vi "thermal_optical_camera_3.vi"() -> ()   [LabVIEW 2025]
panel:
  in  "Stop (F)":bool
  in  "Acquisition Control:\nExposure Time [100, 3E7]":dbl=999.0 caption="Acquisition Control::Exposure Time" min=100.0 max=29999995.0
  in  "Analog Control:\nGain [0, 27]":dbl caption="Analog Control::Gain" min=0.0 max=27.045663671679687
  in  "Analog Control:\nBlack Level [-5, 10]":dbl caption="Analog Control::Black Level" min=-5.0000011920928955 max=10.000002384185791
  in  "Analog Control:\nGamma [0.25, 4.00]":dbl=0.800048828125 caption="Analog Control::Gamma" min=0.25 max=4.0 step=0.05
  out "Optical camera":T1(plugin-control)
  in  "optical capture interval (s)":dbl
  in  "File Path":string="C:\\Digambar\\Metal_thin_wall\\Optical_images\\Optical_images"
  out "File Name Out":string
  out "Frames":i32
  in  "thermal capture interval (s)":dbl
  out "Thermal camera":T1(plugin-control)
  out "Output":string
  in  "Flag Button":bool
  in  "Stop & Save":bool
  in  "Stop Preview":bool
  in  "Focus":dbl(slide) scale=0.0..100.0
  in  "Record":bool
  # "(1) Run VI"
  # "(2) After thermal camera calibration message (in terminal), press START"
  # "(3) Stop & Save"
  # "Destination for Optical Images:"
  # "(Enter \"28\")"
  # "Thermal Record"
  # "change folder names each time you run,\nso it saves data sets in dedicated folders:\nfolder1\nfolder2\nfolder3\netc..."
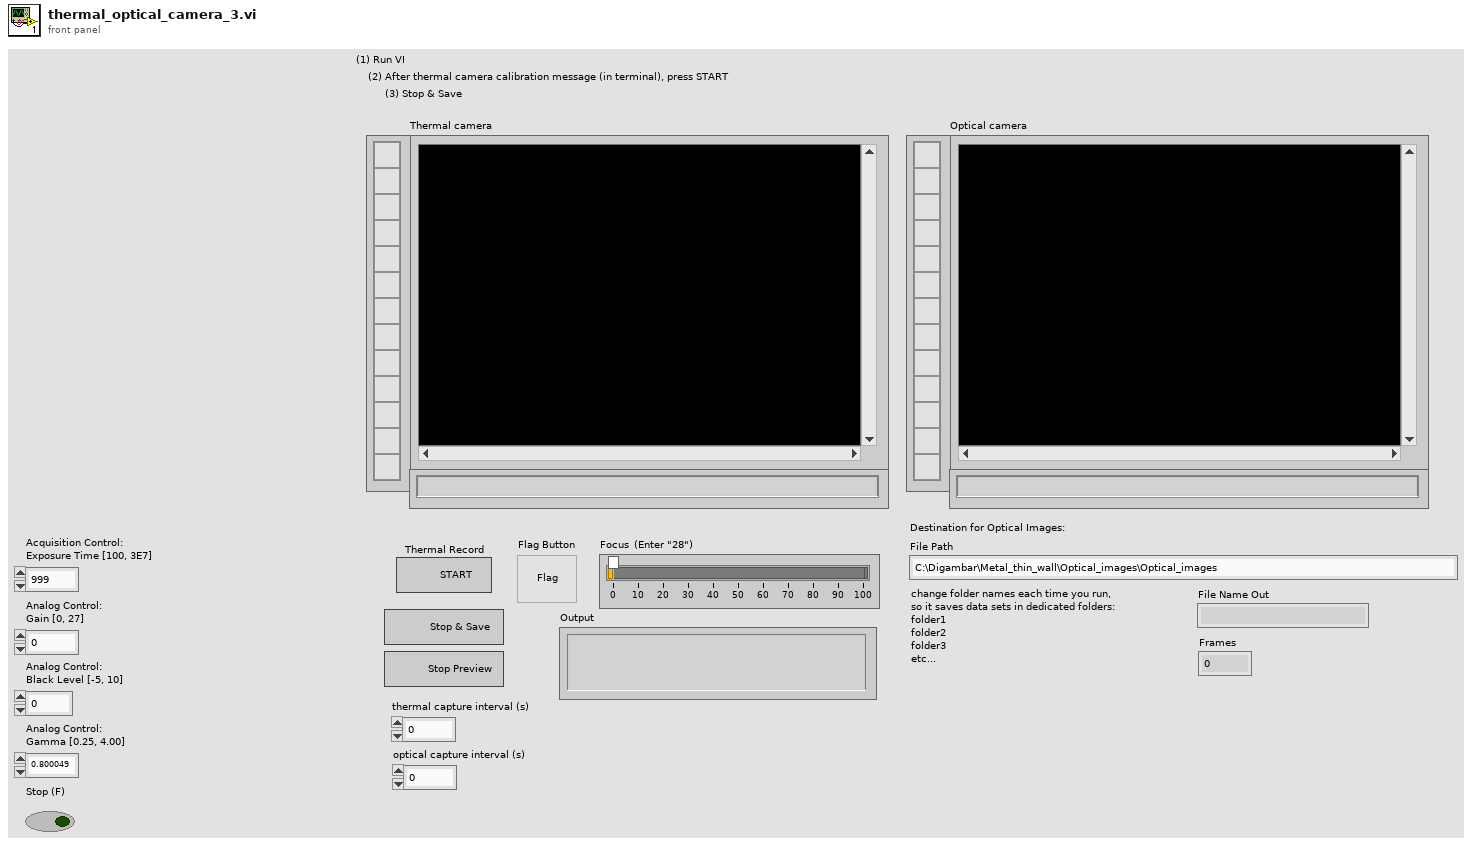
[diagram p1: front panel]
types:
  T1 = typedef "IMAQ Image.ctl" = refnum<image>
  T2 = enum16{"Standard", "Buffered", "CRLF", "Immediate"}
  T3 = enum16{"open", "replace", "create", "open or create", "replace or create", "replace or create with confirmation"}
  T4 = enum16{"big-endian, network order", "native, host order", "little-endian"}
  T5 = typedef "Image Type" = u32
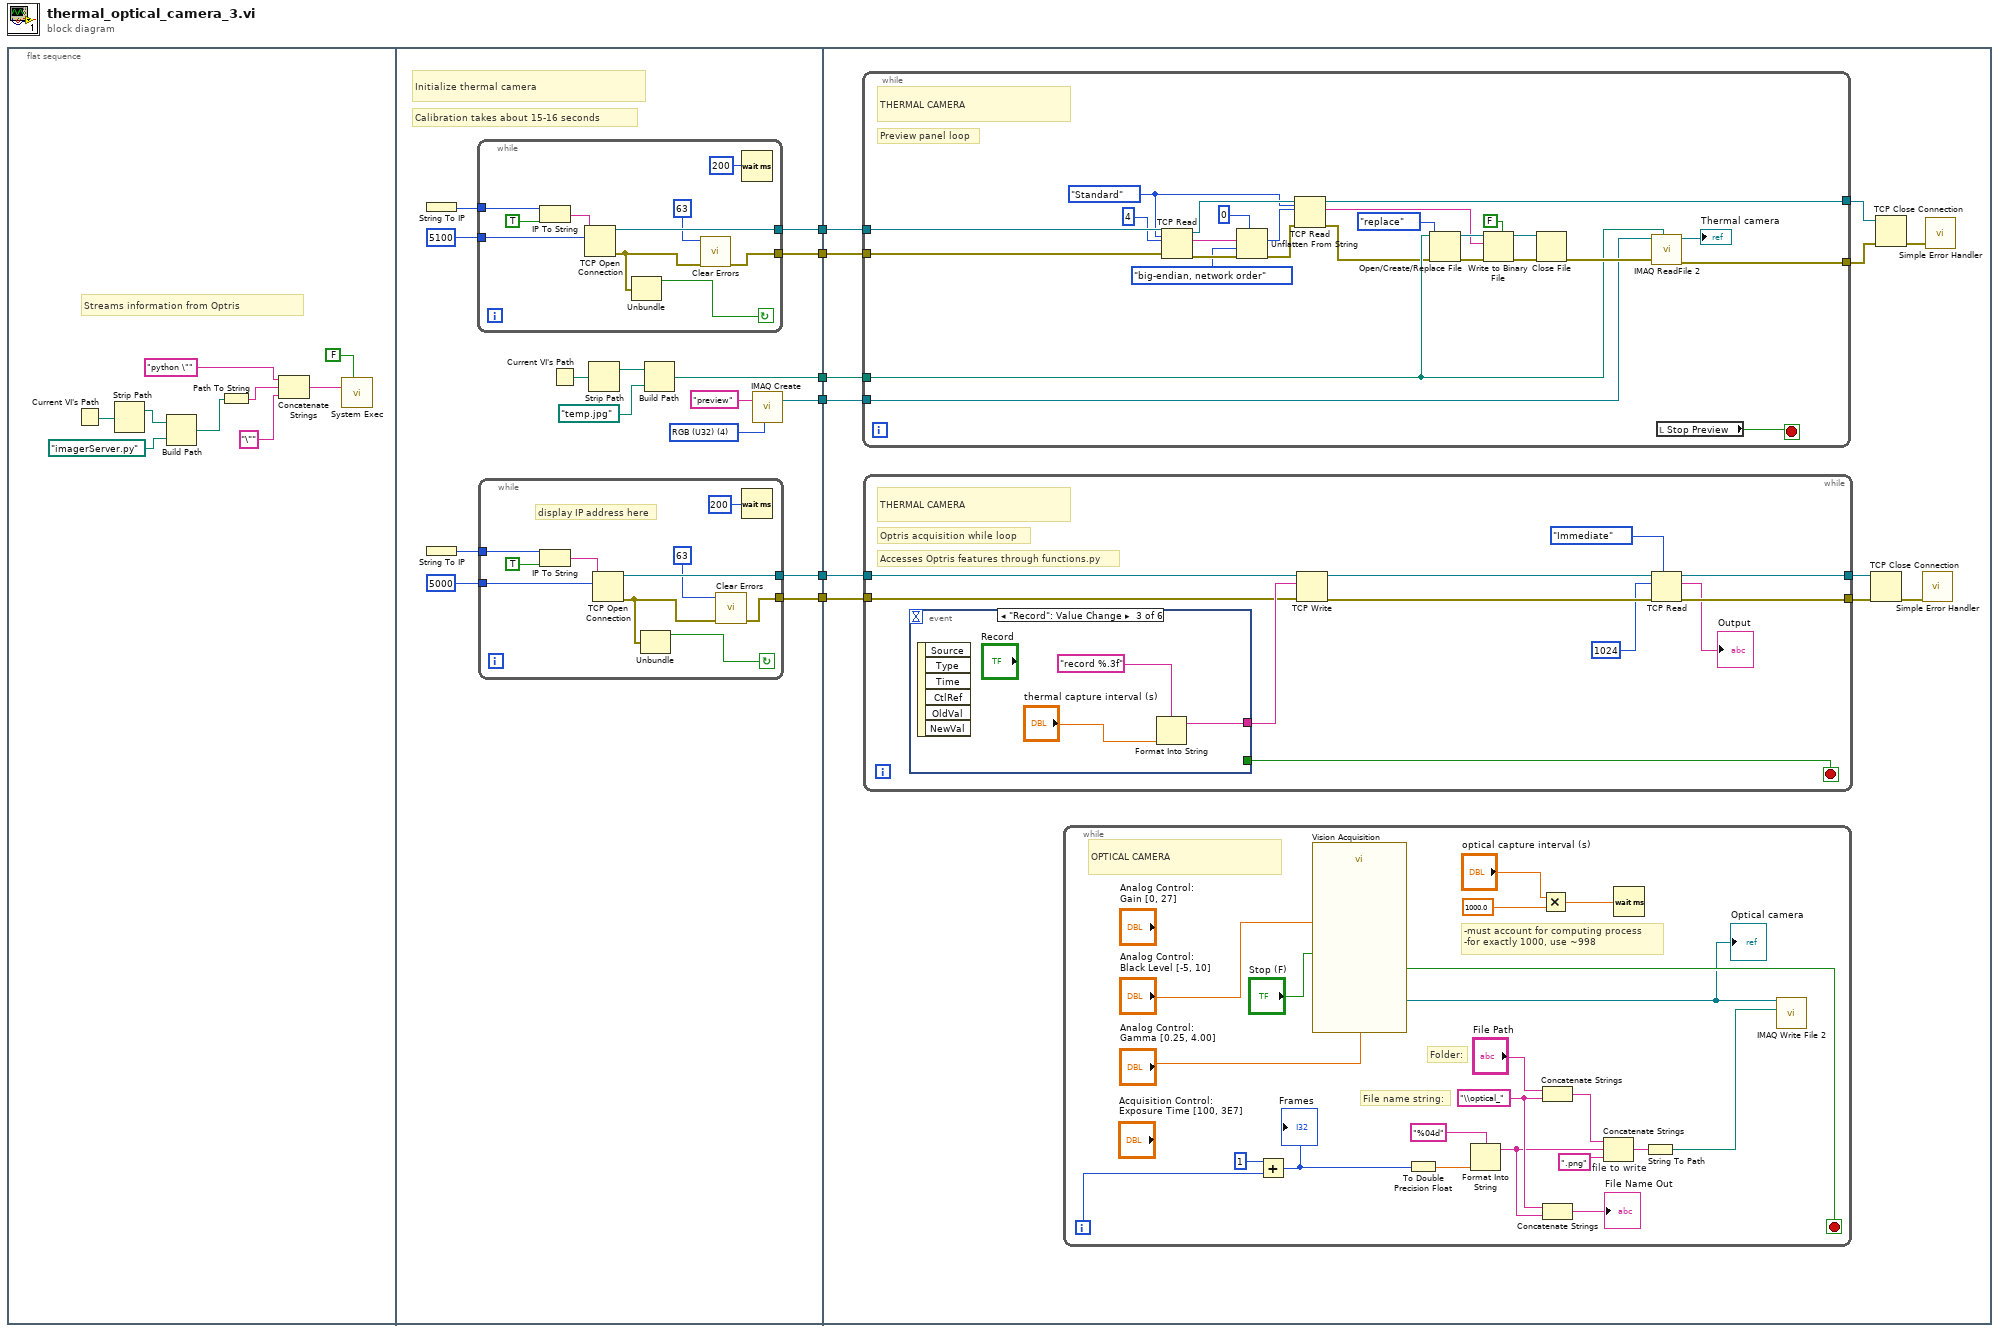
[diagram p0: block diagram]
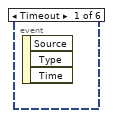
[diagram p2: hidden frame]
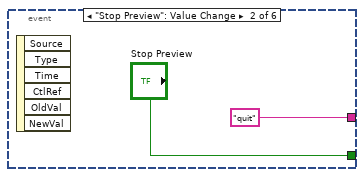
[diagram p3: hidden frame]
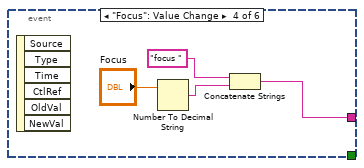
[diagram p4: hidden frame]
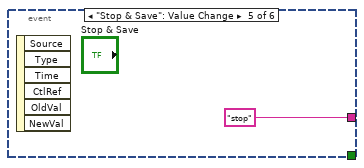
[diagram p5: hidden frame]
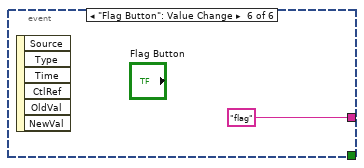
[diagram p6: hidden frame]
diagram:
  n1 = flat-sequence {
    tunnel: [w21] -> w6
    tunnel: [w20] -> w5
    tunnel: [w19] -> w4
    tunnel: [w18] -> w3
    tunnel: [w17] -> w2
    tunnel: [w16] -> w1
    tunnel: w1 -> [w56]
    tunnel: w2 -> [w57]
    tunnel: w3 -> [w52]
    tunnel: w4 -> [w51]
    tunnel: w5 -> [w58]
    tunnel: w6 -> [w59]
    frame #0 {
      # "Streams information from Optris"
      n2 = Current VI's Path() -> (path=w10:path)
      n3 = Strip Path(path=w10) -> (stripped path=w11:path)  [unwired: 1 out]
      n4 = Build Path(base path=w11, name or relative path=path "imagerServer.py") -> (appended path=w8:path)
      n5 = Path To String(path=w8) -> (string=w14:string)
      n6 = Concatenate Strings("python \"" ("string"), w14, "\"" ("string")) -> (w13:string)
      n7 = call <vilib>:"System Exec.vi"("wait until completion? (T)"=FALSE, "command line"=w13) -> ()  [unwired: 6 in, 4 out]
    }
    frame #1 {
      w22 = T5 4 items=["Grayscale (U8)", "Grayscale (I16)", "Grayscale (SGL)", "Complex (CSG)", "RGB (U32)", "HSL (U32)", "RGB (U64)", "Grayscale (U16)"] ("Image Type")
      # "Initialize thermal camera"
      # "Calibration takes about 15-16 seconds"
      n8 = String To IP() -> (0:w30:u32)  [unwired: 1 in]
      n9 = String To IP() -> (0:w29:u32)  [unwired: 1 in]
      n10 = while {
        tunnel: w30 -> [w40]
        tunnel: [w34] -> w21
        tunnel: [w38] -> w20
        tunnel: u16 5100 ("remote port or service name") -> [w36]
        stop <- w31 continue-if-true
        n11 = IP To String(1:TRUE ("dot notation? (F)"), 2:w40) -> (0:w39:string)
        n12 = TCP Open Connection(address=w39, remote port or service name=w36) -> (connection ID=w38:refnum<k5>, error out=w35:errorcluster)  [unwired: 3 in]
        n13 = Unbundle(w35) -> ("status"=w31:bool)  [unwired: 2 out]
        n14 = call <vilib>:"Clear Errors.vi"("error in (no error)"=w35, "specific error code to clear (0: all)"=63) -> ("error out"=w34:errorcluster)  [unwired: 4 in, 1 out]
        n15 = Wait (ms)(milliseconds to wait=u32 200) -> ()  [unwired: 1 out]
      }
      n16 = while {
        tunnel: [w44] -> w19
        tunnel: [w50] -> w18
        tunnel: w29 -> [w48]
        tunnel: u16 5000 ("remote port or service name") -> [w46]
        stop <- w41 continue-if-true
        # "display IP address here"
        n17 = IP To String(1:TRUE ("dot notation? (F)"), 2:w48) -> (0:w49:string)
        n18 = TCP Open Connection(address=w49, remote port or service name=w46) -> (connection ID=w50:refnum<k5>, error out=w45:errorcluster)  [unwired: 3 in]
        n19 = Unbundle(w45) -> ("status"=w41:bool)  [unwired: 2 out]
        n20 = call <vilib>:"Clear Errors.vi"("error in (no error)"=w45, "specific error code to clear (0: all)"=63) -> ("error out"=w44:errorcluster)  [unwired: 4 in, 1 out]
        n21 = Wait (ms)(milliseconds to wait=u32 200) -> ()  [unwired: 1 out]
      }
      n22 = Current VI's Path() -> (path=w28:path)
      n23 = Strip Path(path=w28) -> (stripped path=w27:path)  [unwired: 1 out]
      n24 = Build Path(base path=w27, name or relative path=path "temp.jpg") -> (appended path=w17:path)
      n25 = call "IMAQ Create"("Image Name"="preview", "Image Type"=w22) -> ("New Image"=w16:T1)  [unwired: 3 in, 1 out]
    }
    frame #2 {
      n26 = while {
        tunnel: [w129] -> w61
        tunnel: [w131] -> w62
        tunnel: w59 -> [w126]
        tunnel: w58 -> [w125]
        tunnel: w57 -> [w128]
        tunnel: w56 -> [w124]
        stop <- w127 stop-if-true
        w116 = T2."Standard" ("mode (standard)")
        # "THERMAL CAMERA"
        # "Preview panel loop"
        n27 = TCP Read(connection ID=w125, bytes to read=4, error in (no error)=w126, 7:w116) -> (connection ID out=w119:refnum<k5>, data out=w107:string, error out=w122:errorcluster)  [unwired: 1 in]
        n28 = Unflatten From String(type=0, binary string=w107, byte order (0:big-endian, network order)=T4."big-endian, network order", error in (no error)=w122) -> (value=w117:i32, error out=w118:errorcluster)  [unwired: 1 in, 1 out]
        n29 = TCP Read(connection ID=w119, bytes to read=w117, error in (no error)=w118, 7:w116) -> (connection ID out=w131:refnum<k5>, data out=w112:string, error out=w114:errorcluster)  [unwired: 1 in]
        n30 = Open/Create/Replace File(file path (use dialog)=w128, error in=w114, operation (0:open)=T3."replace") -> (refnum out=w113:refnum<file>, error out=w110:errorcluster)  [unwired: 3 in, 1 out]
        n31 = Write to Binary File(file (use dialog)=w113, data=w112, error in=w110, 5:FALSE ("prepend array or string size? (T)")) -> (refnum out=w108:refnum<file>, error out=w109:errorcluster)  [unwired: 2 in, 1 out]
        n32 = Close File(refnum=w108, error in=w109) -> (error out=w130:errorcluster)  [unwired: 1 out]
        n33 = call "IMAQ ReadFile 2"("File Path"=w128, "error in (no error)"=w130, "Image"=w124) -> ("error out"=w129:errorcluster, "Image Out"=→"Thermal camera":T1)  [unwired: 4 in, 3 out]
        n34 = local read "Stop Preview"() -> (w127:bool)
      }
      n35 = while {
        tunnel: [w93] -> w53
        tunnel: [w91] -> w54
        tunnel: w52 -> [w85]
        tunnel: w51 -> [w84]
        stop <- w86 stop-if-true
        # "THERMAL CAMERA"
        # "Optris acquisition while loop"
        # "Accesses Optris features through functions.py"
        n36 = event shown="[2] \"Record\": Value Change" {
          selector: _ -> [_ _ _ _ _ _]
          dyn-events: _ -> [_ _ _ _ _ _]
          timeout: _ -> [_ _ _ _ _ _]
          tunnel: [_ "quit" w99 w101 "stop" "flag"] -> w90
          tunnel: [_ "Stop Preview" _ _ _ _] -> w86
          event Timeout {
            n37 = event-data() -> ()  [unwired: 1 in, 3 out]
          }
          event "Stop Preview": Value Change {
            n38 = event-data() -> ()  [unwired: 1 in, 6 out]
          }
          event "Record": Value Change {
            n39 = event-data() -> ()  [unwired: 1 in, 6 out]
            n40 = Format Into String(format string="record %.3f", "thermal capture interval (s)") -> (resulting string=w99:string)  [unwired: 2 in, 1 out]
          }
          event "Focus": Value Change {
            n41 = event-data() -> ()  [unwired: 1 in, 6 out]
            n42 = Number To Decimal String(number="Focus") -> (decimal integer string=w103:string)  [unwired: 1 in]
            n43 = Concatenate Strings("focus ", w103) -> (w101:string)
          }
          event "Stop & Save": Value Change {
            n44 = event-data() -> ()  [unwired: 1 in, 6 out]
          }
          event "Flag Button": Value Change {
            n45 = event-data() -> ()  [unwired: 1 in, 6 out]
          }
        }
        n46 = TCP Write(connection ID=w85, data in=w90, error in (no error)=w84) -> (connection ID out=w92:refnum<k5>, error out=w94:errorcluster)  [unwired: 1 in, 1 out]
        n47 = TCP Read(connection ID=w92, bytes to read=1024, error in (no error)=w94, 7:T2."Immediate" ("mode (standard)")) -> (connection ID out=w91:refnum<k5>, data out=→"Output":string, error out=w93:errorcluster)  [unwired: 1 in]
      }
      n48 = while {
        i -> [w64]
        stop <- w82 stop-if-true
        w70 = "\\optical_" ("string")
        # "-must account for computing process\n-for exactly 1000, use ~998"
        # "OPTICAL CAMERA"
        # "Folder:"
        # "File name string:"
        n49 = Add(x=1, y=w64) -> (x+y=w63:i32)
        "Frames" <- w63
        n50 = call "Vision Acquisition"("Analog Control::Black Level"="Analog Control:\nBlack Level [-5, 10]", "Analog Control::Gamma"="Analog Control:\nGamma [0.25, 4.00]", "Stop (F)"="Stop (F)") -> ("Image Out"=w81:T1, "Stopped"=w82:bool)  [unwired: 22 in, 1 out]
        "Optical camera" <- w81
        n51 = To Double Precision Float(number=w63) -> (double precision float=w66:dbl)
        n52 = Format Into String(format string="%04d" ("time format string (%c)"), w66) -> (resulting string=w68:string)  [unwired: 2 in, 1 out]
        n53 = Multiply(x="optical capture interval (s)", y=1000.0) -> (x*y=w76:dbl)
        n54 = Concatenate Strings("File Path", w70) -> (w71:string)
        n55 = Concatenate Strings(w70, w68) -> (→"File Name Out":string)
        n56 = Concatenate Strings "file to write"(w71, w68, ".png" ("string")) -> (w78:string)
        n57 = Wait (ms)(milliseconds to wait=w76) -> ()  [unwired: 1 out]
        n58 = String To Path(string=w78) -> (path=w74:path)
        n59 = call-poly "IMAQ Write File 2"("File Path"=w74, "Image"=w81) -> ()  [unwired: 8 in, 2 out]
      }
      n60 = TCP Close Connection(connection ID=w54, error in (no error)=w53) -> (error out=w55:errorcluster)  [unwired: 1 in, 1 out]
      n61 = TCP Close Connection(connection ID=w62, error in (no error)=w61) -> (error out=w60:errorcluster)  [unwired: 1 in, 1 out]
      n62 = call <vilib>:"Simple Error Handler.vi"("error in (no error)"=w55) -> ()  [unwired: 4 in, 5 out]
      n63 = call <vilib>:"Simple Error Handler.vi"("error in (no error)"=w60) -> ()  [unwired: 4 in, 5 out]
    }
  }
